vi "Joysticks.vi"(9 "Mode":enum16{"Init", "Run", "End"}(ring)) -> (0 "GamePad":T1, 1 "Arm Joystick":T3, 2 "Right Driving Joystick Values":T4, 3 "Left Driving Joystick Values":T5)   [LabVIEW 2013]
uses:
  Type Defs/USB Ports.ctl
  <vilib>/Rock Robotics/WPI/Joystick/WPI_JoystickDeviceEnum.ctl
  Type Defs/Left Drive Joystick.ctl
  <vilib>/Rock Robotics/WPI/Joystick/WPI_JoystickButtonState.ctl
  Type Defs/Right Drive Joystick.ctl
  Type Defs/Arm Joystick.ctl
  Type Defs/Gamepad.ctl
panel:
  in  "USB slots":T6={"Left Driving Joystick"=enum."USB 1", "Right Driving Joystick"=enum."USB 2", "Arm Joystick"=enum."USB 3", "Gamepad"=enum."USB 4"}
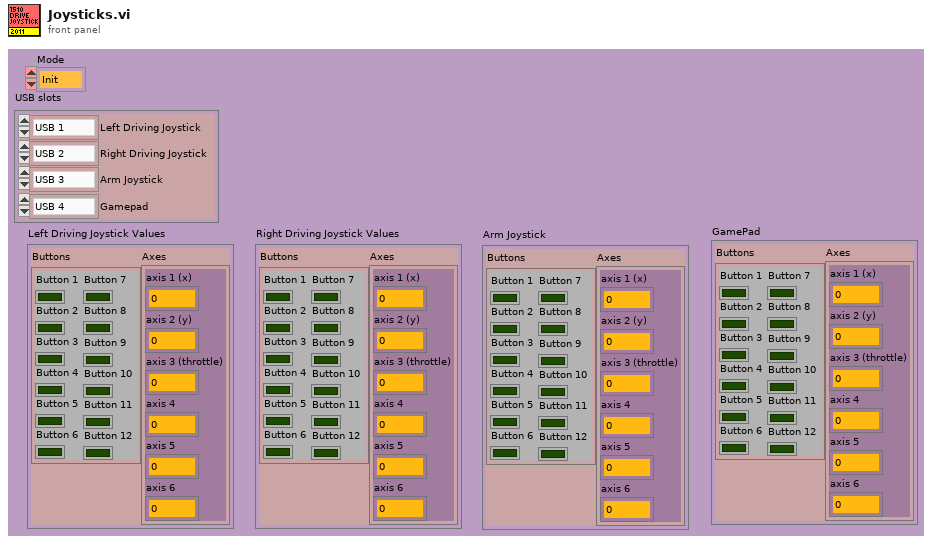
[diagram p1: front panel]
types:
  T1 = typedef "Gamepad.ctl" = cluster{"Buttons":T2, "Axes":cluster{"axis 1 (x)":dbl, "axis 2 (y)":dbl, "axis 3 (throttle)":dbl, "axis 4":dbl, "axis 5":dbl, "axis 6":dbl}}
  T2 = typedef "WPI_JoystickButtonState.ctl" = cluster{"Button 1":bool, "Button 2":bool, "Button 3":bool, "Button 4":bool, "Button 5":bool, "Button 6":bool, "Button 7":bool, "Button 8":bool, "Button 9":bool, "Button 10":bool, "Button 11":bool, "Button 12":bool}
  T3 = typedef "Arm Joystick.ctl" = cluster{"Buttons":T2, "Axes":cluster{"axis 1 (x)":dbl, "axis 2 (y)":dbl, "axis 3 (throttle)":dbl, "axis 4":dbl, "axis 5":dbl, "axis 6":dbl}}
  T4 = typedef "Right Drive Joystick.ctl" = cluster{"Buttons":T2, "Axes":cluster{"axis 1 (x)":dbl, "axis 2 (y)":dbl, "axis 3 (throttle)":dbl, "axis 4":dbl, "axis 5":dbl, "axis 6":dbl}}
  T5 = typedef "Left Drive Joystick.ctl" = cluster{"Buttons":T2, "Axes":cluster{"axis 1 (x)":dbl, "axis 2 (y)":dbl, "axis 3 (throttle)":dbl, "axis 4":dbl, "axis 5":dbl, "axis 6":dbl}}
  T6 = typedef "USB Ports.ctl" = cluster{"Left Driving Joystick":T7, "Right Driving Joystick":T7, "Arm Joystick":T7, "Gamepad":T7}
  T7 = typedef "WPI_JoystickDeviceEnum.ctl" = enum16{"USB 1", "USB 2", "USB 3", "USB 4", "Kinect 1", "Kinect 2"}
  T8 = typedef "WPI_JoystickDevRef.ctl" = cluster{"Device":T7}
  T9 = cluster{"axis 1 (x)":dbl, "axis 2 (y)":dbl, "axis 3 (throttle)":dbl, "axis 4":dbl, "axis 5":dbl, "axis 6":dbl}
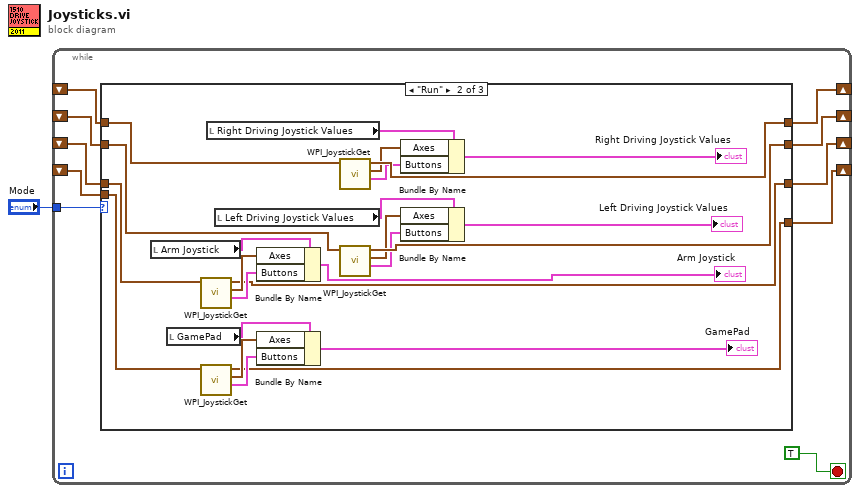
[diagram p0: block diagram]
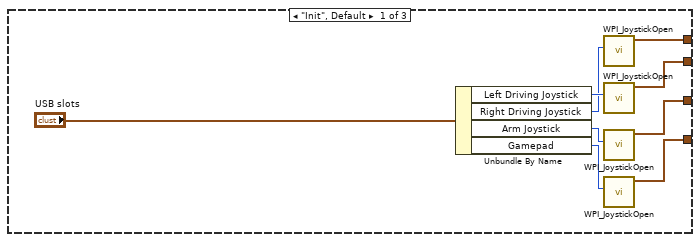
[diagram p2: hidden frame]
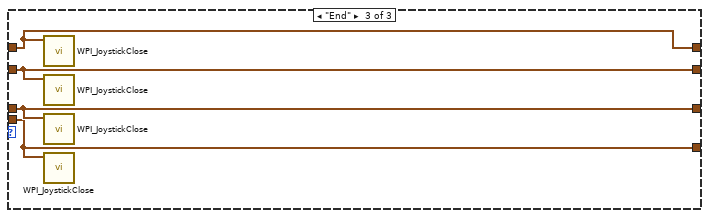
[diagram p3: hidden frame]
diagram:
  n1 = while {
    tunnel: "Mode" -> [w11]
    shift-right: [w10] -> _
    shift-left: _ -> [w7]
    shift-right: [w9] -> _
    shift-left: _ -> [w8]
    shift-right: [w5] -> _
    shift-left: _ -> [w4]
    shift-right: [w3] -> _
    shift-left: _ -> [w2]
    stop <- TRUE stop-if-true
    n2 = case shown="\"Run\"" w11 {
      tunnel: [w18 w41 w48] -> w10
      tunnel: [w16 w42 w47] -> w9
      tunnel: w8 -> [_ w44 w47]
      tunnel: w7 -> [_ w43 w48]
      tunnel: [w14 w29 w46] -> w5
      tunnel: w4 -> [_ w31 w46]
      tunnel: [w13 w23 w45] -> w3
      tunnel: w2 -> [_ w26 w45]
      frame "Init", Default {
        n3 = Unbundle By Name("USB slots") -> ("Left Driving Joystick"=w20:T7, "Right Driving Joystick"=w19:T7, "Arm Joystick"=w15:T7, "Gamepad"=w12:T7)
        n4 = call <vilib>:"WPI_JoystickOpen.vi"("JoystickDevice"=w19) -> ("JoystickDevRef"=w16:T8)  [unwired: 10 out]
        n5 = call <vilib>:"WPI_JoystickOpen.vi"("JoystickDevice"=w20) -> ("JoystickDevRef"=w18:T8)  [unwired: 10 out]
        n6 = call <vilib>:"WPI_JoystickOpen.vi"("JoystickDevice"=w15) -> ("JoystickDevRef"=w14:T8)  [unwired: 10 out]
        n7 = call <vilib>:"WPI_JoystickOpen.vi"("JoystickDevice"=w12) -> ("JoystickDevRef"=w13:T8)  [unwired: 10 out]
      }
      frame "Run" {
        n8 = local read "Arm Joystick"() -> (w28:T3)
        n9 = local read "GamePad"() -> (w22:T1)
        n10 = call <vilib>:"WPI_JoystickGet.vi"("JoystickDevRef"=w31) -> ("Buttons"=w32:T2, "Axes"=w30:T9, "JoystickDevRef"=w29:T8)  [unwired: 1 in, 3 out]
        n11 = call <vilib>:"WPI_JoystickGet.vi"("JoystickDevRef"=w26) -> ("Buttons"=w24:T2, "Axes"=w25:T9, "JoystickDevRef"=w23:T8)  [unwired: 1 in, 3 out]
        n12 = local read "Right Driving Joystick Values"() -> (w33:T4)
        n13 = local read "Left Driving Joystick Values"() -> (w34:T5)
        n14 = Bundle By Name(cluster=w28, "Axes"=w30, "Buttons"=w32) -> (→"Arm Joystick":T3)
        n15 = Bundle By Name(cluster=w22, "Axes"=w25, "Buttons"=w24) -> (→"GamePad":T1)
        n16 = call <vilib>:"WPI_JoystickGet.vi"("JoystickDevRef"=w44) -> ("Buttons"=w39:T2, "Axes"=w40:T9, "JoystickDevRef"=w42:T8)  [unwired: 1 in, 3 out]
        n17 = call <vilib>:"WPI_JoystickGet.vi"("JoystickDevRef"=w43) -> ("Buttons"=w37:T2, "Axes"=w38:T9, "JoystickDevRef"=w41:T8)  [unwired: 1 in, 3 out]
        n18 = Bundle By Name(cluster=w33, "Axes"=w40, "Buttons"=w39) -> (→"Right Driving Joystick Values":T4)
        n19 = Bundle By Name(cluster=w34, "Axes"=w38, "Buttons"=w37) -> (→"Left Driving Joystick Values":T5)
      }
      frame "End" {
        n20 = call <vilib>:"WPI_JoystickClose.vi"("JoystickDevRef"=w47) -> ()  [unwired: 11 out]
        n21 = call <vilib>:"WPI_JoystickClose.vi"("JoystickDevRef"=w48) -> ()  [unwired: 11 out]
        n22 = call <vilib>:"WPI_JoystickClose.vi"("JoystickDevRef"=w46) -> ()  [unwired: 11 out]
        n23 = call <vilib>:"WPI_JoystickClose.vi"("JoystickDevRef"=w45) -> ()  [unwired: 11 out]
      }
    }
  }
